vi "CLD 7 Time Stamp to String Challenge Exercise.vi"(8 "Fehler (Eingang)":T2) -> (0 "Fehler (Ausgang)":T2, 3 "Code-String (Ausgang)":string)   [LabVIEW 2014]
doc: "CLD-Übung 7"
uses:
  <vilib>/Utility/miscctls.llb/LVDateTimeRec.ctl
panel:
  out "Datum/Zeit":T1
  in  "in Weltzeit (F)":bool
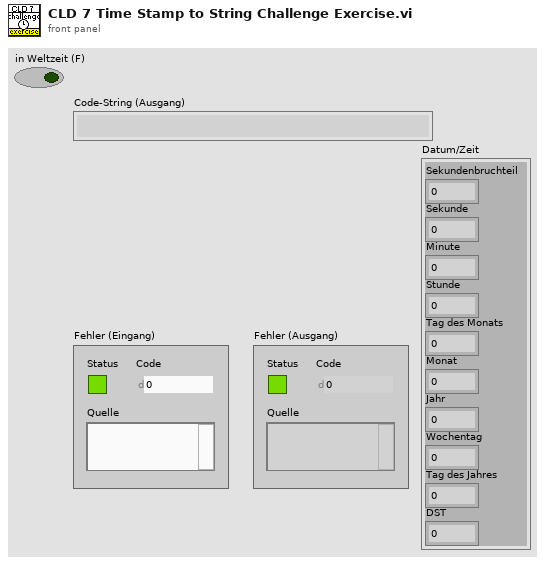
[diagram p1: front panel]
types:
  T1 = typedef "LVDateTimeRec.ctl" = cluster{"fractional second":dbl, "second":i32, "minute":i32, "hour":i32, "day of month":i32, "month":i32, "year":i32, "day of week":i32, "day of year":i32, "DST":i32}
  T2 = cluster{"Status":bool, "Code":i32, "Quelle":string}
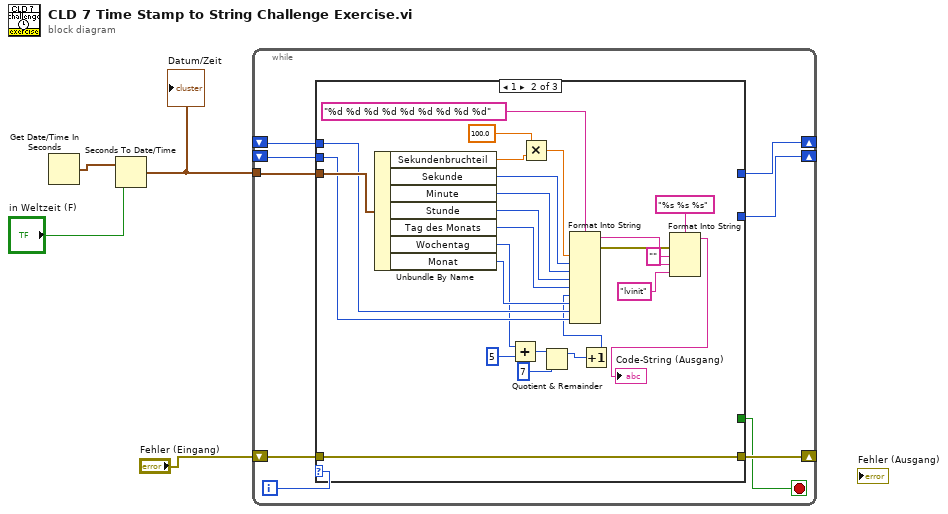
[diagram p0: block diagram]
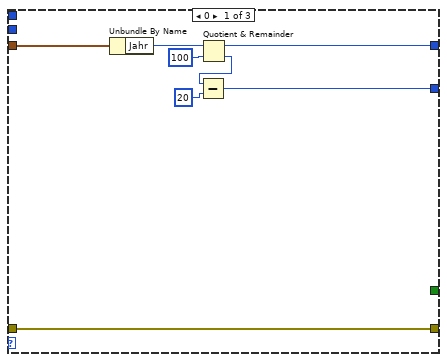
[diagram p2: hidden frame]
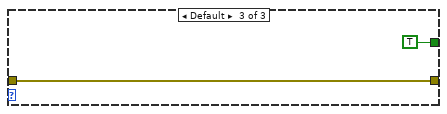
[diagram p3: hidden frame]
diagram:
  n1 = Get Date/Time In Seconds() -> (seconds since 1Jan1904=w3:timestamp)
  n2 = Seconds To Date/Time(time stamp (now)=w3, to UTC (F)="in Weltzeit (F)") -> (date time rec=w1:T1)
  "Datum/Zeit" <- w1
  n3 = while {
    shift-right: [w11] -> _
    shift-left: "Fehler (Eingang)" -> [w12]
    tunnel: w1 -> [w10]
    shift-right: [w8] -> _
    shift-left: _ -> [w7]
    shift-right: [w9] -> _
    shift-left: _ -> [w6]
    i -> [w13]
    stop <- w5 stop-if-true
    n4 = case shown="1" w13 {
      tunnel: w12 -> [w21 w46 w48]
      tunnel: [w21 w46 w48] -> w11
      tunnel: w10 -> [w20 w36 _]
      tunnel: [w15 _ _] -> w9
      tunnel: [w14 _ _] -> w8
      tunnel: w7 -> [_ w31 _]
      tunnel: w6 -> [_ w30 _]
      tunnel: [_ _ TRUE] -> w5
      frame 0 {
        n5 = Unbundle By Name(w20) -> ("Jahr"=w18:i32)
        n6 = Quotient & Remainder(x=w18, y=100) -> (x-y*floor(x/y)=w14:i32, floor(x/y)=w17:i32)
        n7 = Subtract(x=w17, y=20) -> (x-y=w15:i32)
      }
      frame 1 {
        n8 = Unbundle By Name(w36) -> ("Sekundenbruchteil"=w35:dbl, "Sekunde"=w45:i32, "Minute"=w44:i32, "Stunde"=w43:i32, "Tag des Monats"=w42:i32, "Wochentag"=w27:i32, "Monat"=w32:i32)
        n9 = Add(x=w27, y=5) -> (x+y=w25:i32)
        n10 = Multiply(x=100.0, y=w35) -> (x*y=w33:dbl)
        n11 = Quotient & Remainder(x=w25, y=7) -> (x-y*floor(x/y)=w23:i32)  [unwired: 1 out]
        n12 = Increment(x=w23) -> (x+1=w22:i32)
        n13 = Format Into String(format string="%d %d %d %d %d %d %d %d %d" ("Format-String"), w33, w45, w44, w43, w42, w22, w32, w31, w30) -> (resulting string=w39:string, error out=w37:errorcluster)  [unwired: 2 in]
        n14 = Format Into String(format string="%s %s %s" ("Format-String"), error in=w37, "" ("Eingang 1"), w39, "lvinit" ("Eingang 3")) -> (resulting string=→"Code-String (Ausgang)":string)  [unwired: 1 in, 1 out]
      }
      frame Default {
      }
    }
  }
